vi "Panel Split Engine Example.vi"() -> ()   [LabVIEW 2016]
uses:
  PanelRootNode/PanelRootNode.lvclass
  QueueManager.llb/Destroy.vi
  QueueManager.llb/Remove.vi
  PanelDataNode/PanelDataNode.lvclass
  QueueManager.llb/CreatQueue.vi
  <vilib>/Utility/error.llb/DialogType.ctl
  PanelExample.lvclass
panel:
  out "SelfNode*":refnum<data-value>
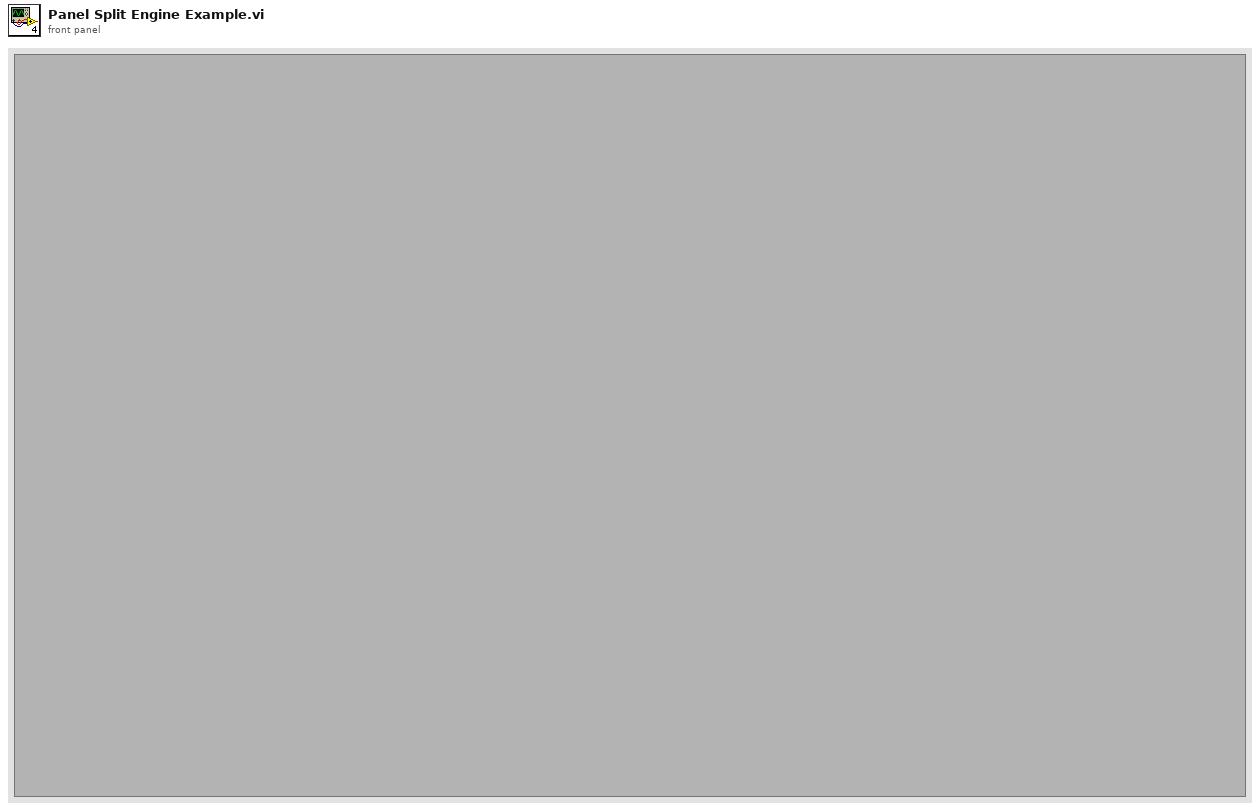
[diagram p1: front panel]
types:
  T1 = cluster{"error":errorcluster, "Event":string, "Data":variant, "Q_Local":string, "RootNode*":refnum<data-value>, "Caller":string}
  T2 = typedef "DialogType.ctl" = u16
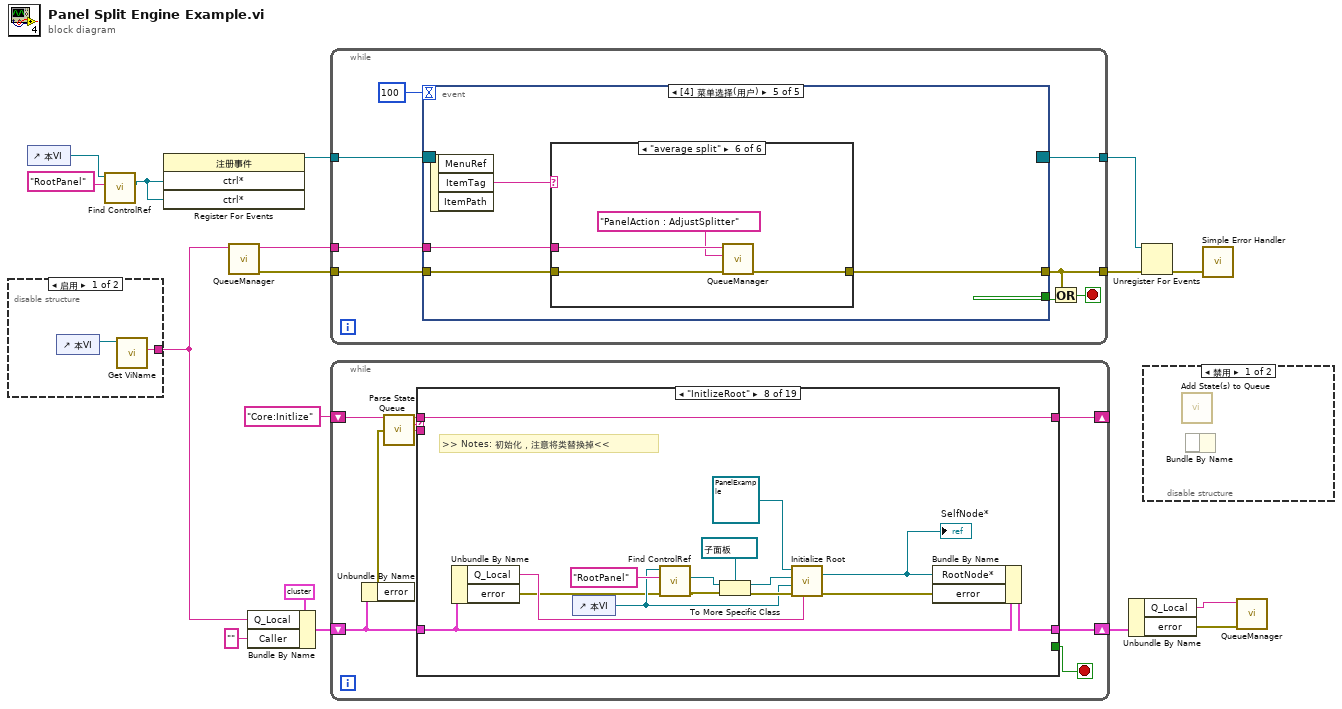
[diagram p0: block diagram]
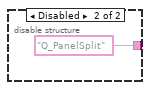
[diagram p2: hidden frame]
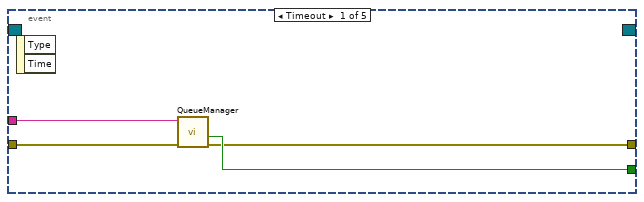
[diagram p4: hidden frame]
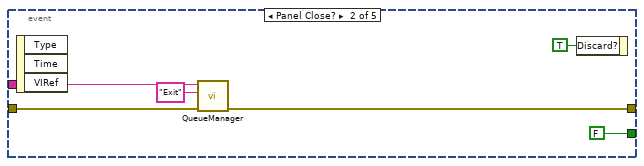
[diagram p5: hidden frame]
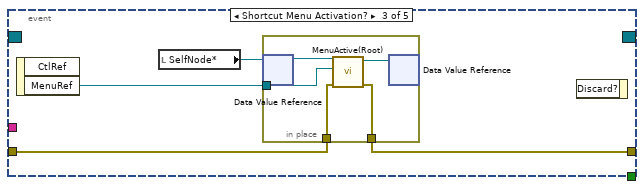
[diagram p6: hidden frame]
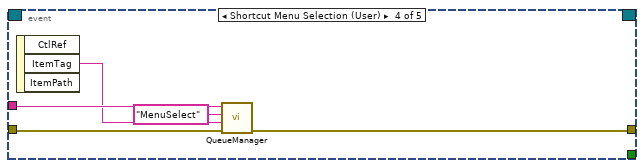
[diagram p7: hidden frame]
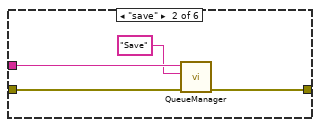
[diagram p9: hidden frame]
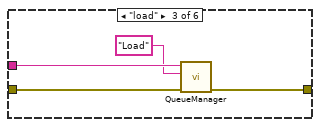
[diagram p10: hidden frame]
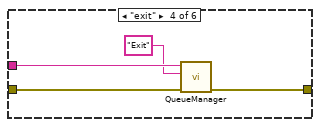
[diagram p11: hidden frame]
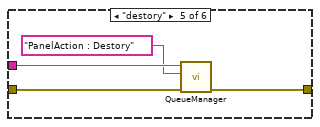
[diagram p12: hidden frame]
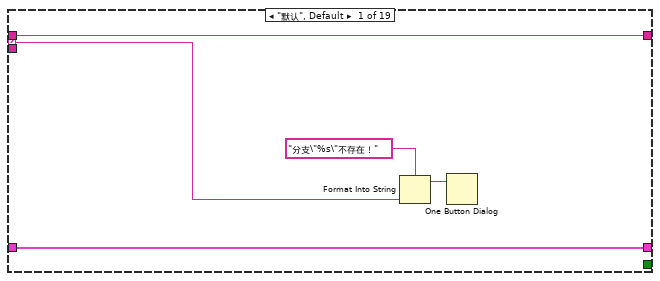
[diagram p13: hidden frame]
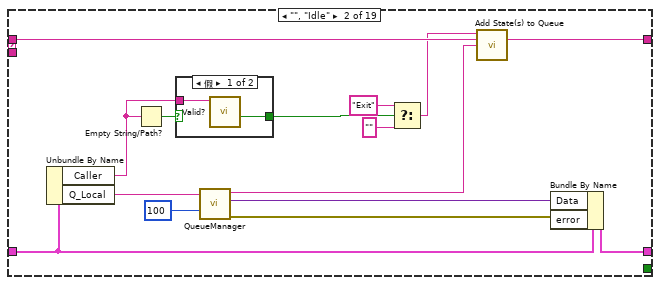
[diagram p14: hidden frame]
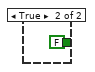
[diagram p15: hidden frame]
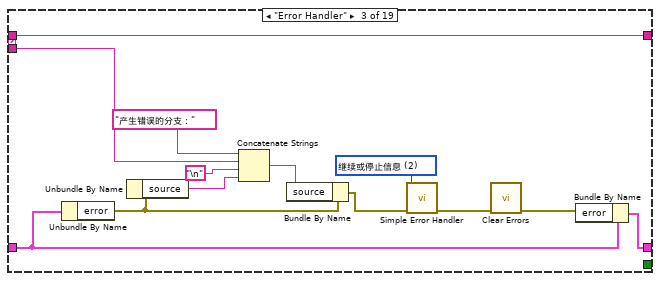
[diagram p16: hidden frame]
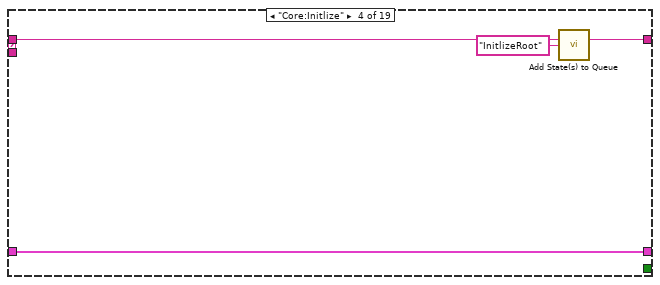
[diagram p17: hidden frame]
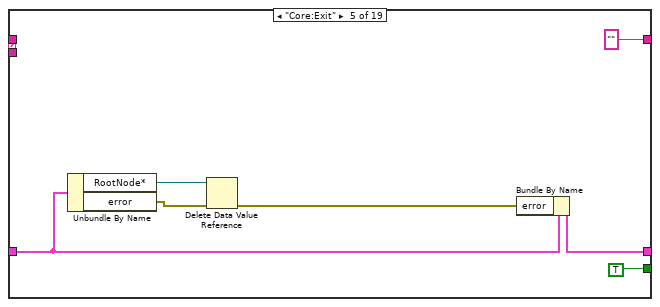
[diagram p18: hidden frame]
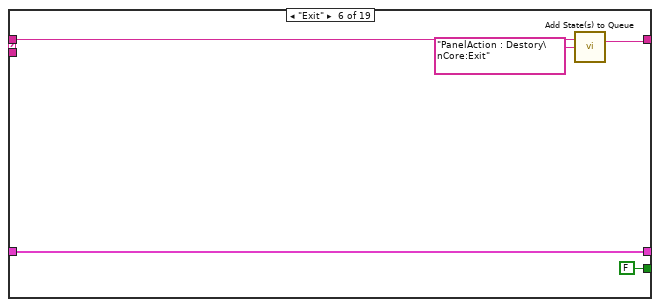
[diagram p19: hidden frame]
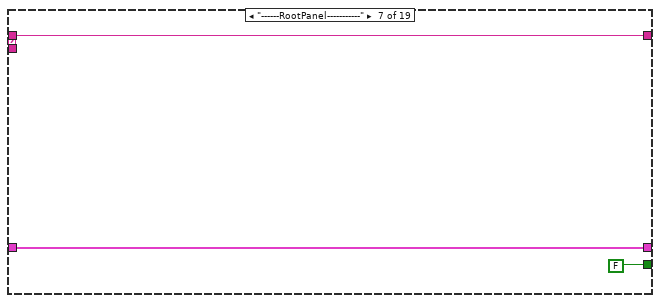
[diagram p20: hidden frame]
diagram:
  n1 = disable-structure shown="启用" {
    disable-tunnel: [w17 "Q_PanelSplit" ("QueueName")] -> w8
    frame Enabled {
      n2 = control-ref of="本VI"() -> (w18:refnum<vi>)
      n3 = call "Get ViName.vi"("VI*"=w18) -> ("VI Name"=w17:string)  [unwired: 8 in, 2 out]
    }
    frame Disabled {
    }
  }
  n4 = control-ref of="本VI"() -> (w6:refnum<vi>)
  n5 = call "Find ControlRef.vi"("control name"="RootPanel", "vi*"=w6) -> ("ctrl*"=w4:refnum<vi>)  [unwired: 7 in, 2 out]
  n6 = register-events(w4, w4) -> (reference out=w9:refnum<event-registration>)  [unwired: 2 in, 1 out]
  n7 = call-poly "QueueManager.vi"("QueueName"=w8) -> ("error out"=w16:errorcluster)  [unwired: 9 in, 1 out]
  n8 = Bundle By Name(cluster=T1 {"error"={"status"=FALSE, "code"=0, "source"=""}, "Event"="", "Data"=variant, "Q_Local"="", "RootNode*"=refnum, "Caller"=""} ("TmpData"), "Q_Local"=w8, "Caller"="") -> (w11:T1)
  n9 = while {
    tunnel: w16 -> [w26]
    tunnel: w8 -> [w27]
    tunnel: [w23] -> w3
    tunnel: w9 -> [w21]
    tunnel: [w20] -> w1
    stop <- w24 stop-if-true
    n10 = event shown="[4] 菜单选择(用户)" {
      selector: w21 -> [_ _ _ _ _]
      dyn-events: [_ _ _ _ _] -> w20
      timeout: 100 -> [_ _ _ _ _]
      tunnel: [w29 FALSE _ _ _] -> w25
      tunnel: w27 -> [w31 w36 _ w51 w54]
      tunnel: w26 -> [w30 w35 w40 w50 w53]
      tunnel: [w28 w34 w41 w49 w52] -> w23
      event Timeout {
        n11 = event-data() -> ()  [unwired: 1 in, 2 out]
        n12 = call-poly "QueueManager.vi"("error in (no error)"=w30, "Queue Name(unamed)"=w31) -> ("error out"=w28:errorcluster, "Not Exist?"=w29:bool)  [unwired: 8 in]
      }
      event Panel Close? {
        n13 = event-data() -> ()  [unwired: 1 in, 3 out]
        n14 = call-poly "QueueManager.vi"("error in"=w35, "Event"="Exit", "QueueName"=w36) -> ("error out"=w34:errorcluster)  [unwired: 7 in, 1 out]
        n15 = event-data("Discard?"=TRUE ("放弃？")) -> ()  [unwired: 1 in, 1 out]
      }
      event Shortcut Menu Activation? {
        n16 = event-data() -> ("MenuRef"=w39:refnum<k9>)  [unwired: 1 in, 1 out]
        n17 = local read "SelfNode*"() -> (w38:refnum<data-value>)
        n18 = in-place {
          in-place-border: w39 -> [w44]
          in-place-border: w40 -> [w43]
          in-place-border: [w42] -> w41
          n19 = in-place-dvr #1(w38) -> (w46:refnum<class "PanelRootNode.lvclass">)  [unwired: 1 out]
          n20 = call "MenuActive(Root).vi"("error in (no error)"=w43, "菜单引用"=w44, "PanelDataNode 输入"=w46) -> ("error out"=w42:errorcluster, "PanelDataNode 输出"=w45:refnum<class "PanelRootNode.lvclass">)  [unwired: 7 in]
          n21 = in-place-dvr #1(w45) -> ()  [unwired: 2 out]
        }
        n22 = event-data() -> ()  [unwired: 2 in, 1 out]
      }
      event Shortcut Menu Selection (User) {
        n23 = event-data() -> ("ItemTag"=w48:string)  [unwired: 1 in, 2 out]
        n24 = call-poly "QueueManager.vi"("error in"=w50, "Data"=w48, "Event"="MenuSelect", "QueueName"=w51) -> ("error out"=w49:errorcluster)  [unwired: 6 in, 1 out]
      }
      event Menu Selection (User) {
        n25 = event-data() -> ("ItemTag"=w55:string)  [unwired: 1 in, 2 out]
        n26 = case shown="\"average split\"" w55 {
          tunnel: w54 -> [_ w60 w64 w68 w72 w76]
          tunnel: w53 -> [w56 w58 w62 w66 w70 w74]
          tunnel: [w56 w57 w61 w65 w69 w73] -> w52
          frame "假", Default {
          }
          frame "save" {
            n27 = call-poly "QueueManager.vi"("error in"=w58, "Event"="Save", "QueueName"=w60) -> ("error out"=w57:errorcluster)  [unwired: 7 in, 1 out]
          }
          frame "load" {
            n28 = call-poly "QueueManager.vi"("error in"=w62, "Event"="Load", "QueueName"=w64) -> ("error out"=w61:errorcluster)  [unwired: 7 in, 1 out]
          }
          frame "exit" {
            n29 = call-poly "QueueManager.vi"("error in"=w66, "Event"="Exit", "QueueName"=w68) -> ("error out"=w65:errorcluster)  [unwired: 7 in, 1 out]
          }
          frame "destory" {
            n30 = call-poly "QueueManager.vi"("error in"=w70, "Event"="PanelAction : Destory", "QueueName"=w72) -> ("error out"=w69:errorcluster)  [unwired: 7 in, 1 out]
          }
          frame "average split" {
            n31 = call-poly "QueueManager.vi"("error in"=w74, "Event"="PanelAction : AdjustSplitter", "QueueName"=w76) -> ("error out"=w73:errorcluster)  [unwired: 7 in, 1 out]
          }
        }
      }
    }
    n32 = Or(x=w23, y=w25) -> (x .or. y?=w24:bool)
  }
  n33 = while {
    shift-right: [w78] -> w13
    shift-left: w11 -> [w79]
    shift-right: [w77] -> _
    shift-left: "Core:Initlize" -> [w85]
    stop <- w81 stop-if-true
    n34 = Unbundle By Name(w79) -> ("error"=w80:errorcluster)
    n35 = call "Parse State Queue.vi"("State Queue"=w85, "Error In (no error)"=w80) -> ("Remaining States"=w84:string, "Current State"=w83:string, "Arguments"=w82:string)  [unwired: 10 in, 1 out]
    n36 = case shown="\"InitlizeRoot\"" w83 {
      selector: w83 -> [w86 _ _ _ _ _ _ _ _ _ _ _ _ _ _ _ _ _ _]
      tunnel: w84 -> [w89 w101 w121 w124 _ w137 w138 w155 w163 w184 w196 w207 w214 w225 w235 w245 w255 w261 w273]
      tunnel: w82 -> [_ _ w109 _ _ _ _ _ _ _ _ _ _ _ _ _ _ _ _]
      tunnel: [_ _ _ _ TRUE FALSE FALSE _ _ _ _ _ _ _ _ _ _ _ _] -> w81
      tunnel: w79 -> [w90 w98 w111 w125 w128 w134 w139 w148 w165 w182 w200 w206 w213 w223 w233 w243 w253 w260 w271]
      tunnel: [w90 w104 w110 w125 w127 w134 w139 w150 w164 w181 w199 w206 w212 w222 w232 w242 w252 w260 w270] -> w78
      tunnel: [w89 w100 w121 w123 "" ("Remaining States") w136 w138 w155 w163 w184 w195 w207 w214 w225 w235 w245 w255 w261 w273] -> w77
      frame "默认", Default {
        n37 = Format Into String(format string="分支\"%s\"不存在！" ("格式字符串"), w86) -> (resulting string=w88:string)  [unwired: 2 in, 1 out]
        n38 = One Button Dialog(message=w88) -> ()  [unwired: 1 in, 1 out]
      }
      frame "", "Idle" {
        n39 = Unbundle By Name(w98) -> ("Caller"=w92:string, "Q_Local"=w97:string)
        n40 = Empty String/Path?(string/path=w92) -> (empty?=w96:bool)
        n41 = case shown="假" w96 {
          tunnel: [w107 FALSE ("Not Exist?")] -> w95
          tunnel: w92 -> [w106 _]
          frame False {
            n42 = call "Valid?.vi"("Queue Name(unamed)"=w106) -> ("Not Exist?"=w107:bool)  [unwired: 9 in, 1 out]
          }
          frame True {
          }
        }
        n43 = call-poly "QueueManager.vi"("Time out(-1)"=100, "Queue Name"=w97) -> ("error out"=w105:errorcluster, "Data"=w103:variant, "Event"=w102:string)  [unwired: 6 in, 1 out]
        n44 = Select(t="Exit" ("Event"), s=w95, f="") -> (s? t:f=w91:string)
        n45 = call "Add State(s) to Queue.vi"("State(s) in Front (\"\")"=w91, "State(s) in (\"\")"=w101, "State(s) at Back (\"\")"=w102) -> ("States Out"=w100:string)  [unwired: 12 in]
        n46 = Bundle By Name(cluster=w98, "Data"=w103, "error"=w105) -> (w104:T1)
      }
      frame "Error Handler" {
        w118 = T2 2 items=["无对话框", "确定信息", "继续或停止信息", "确定信息＋警告", "继续/停止+警告"] ("type of dialog (OK msg:1)")
        n47 = Unbundle By Name(w111) -> ("error"=w113:errorcluster)
        n48 = Unbundle By Name(w113) -> ("source"=w116:string)
        n49 = Concatenate Strings("产生错误的分支：" ("字符串"), w109, "\n", w116) -> (w114:string)
        n50 = Bundle By Name(cluster=w113, "source"=w114) -> (w112:errorcluster)
        n51 = call <vilib>:"Simple Error Handler.vi"("type of dialog (OK msg:1)"=w118, "error in (no error)"=w112) -> ("error out"=w119:errorcluster)  [unwired: 3 in, 4 out]
        n52 = call <vilib>:"Clear Errors.vi"("error in (no error)"=w119) -> ("error out"=w120:errorcluster)  [unwired: 5 in, 1 out]
        n53 = Bundle By Name(cluster=w111, "error"=w120) -> (w110:T1)
      }
      frame "Core:Initlize" {
        n54 = call "Add State(s) to Queue.vi"("State(s) in (\"\")"=w124, "State(s) at Back (\"\")"="InitlizeRoot" ("State(s) at Back (\"\")")) -> ("States Out"=w123:string)  [unwired: 13 in]
      }
      frame "Core:Exit" {
        n55 = Unbundle By Name(w128) -> ("RootNode*"=w130:refnum<data-value>, "error"=w126:errorcluster)
        n56 = Delete Data Value Reference(data value reference=w130, error in=w126) -> (error out=w129:errorcluster)  [unwired: 1 out]
        n57 = Bundle By Name(cluster=w128, "error"=w129) -> (w127:T1)
      }
      frame "Exit" {
        n58 = call "Add State(s) to Queue.vi"("State(s) in (\"\")"=w137, "State(s) at Back (\"\")"="PanelAction : Destory\nCore:Exit" ("State(s) at Back (\"\")")) -> ("States Out"=w136:string)  [unwired: 13 in]
      }
      frame "------RootPanel-----------" {
      }
      frame "InitlizeRoot" {
        # ">> Notes: 初始化，注意将类替换掉<<"
        n59 = Unbundle By Name(w148) -> ("Q_Local"=w147:string, "error"=w142:errorcluster)
        n60 = control-ref of="本VI"() -> (w143:refnum<vi>)
        n61 = call "Find ControlRef.vi"("error in (no error)"=w142, "control name"="RootPanel", "vi*"=w143) -> ("error out"=w145:errorcluster, "ctrl*"=w144:refnum<vi>)  [unwired: 6 in, 1 out]
        n62 = To More Specific Class(target class=refnum<vi> refnum ("RootPanel"), reference=w144, error in=w145) -> (specific class reference=w153:refnum<vi>, error out=w152:errorcluster)
        n63 = call-dynamic "Initialize Root.vi"("RootQueueName"=w147, "error in (no error)"=w152, "CurrentVi*"=w143, "RootPanel*"=w153, "PanelRootNode 输入"=refnum<class "PanelExample.lvclass"> refnum ("PanelExample.lvclass")) -> ("error out"=w151:errorcluster, "SelfNode*"=w149:refnum<data-value>)  [unwired: 5 in]
        "SelfNode*" <- w149
        n64 = Bundle By Name(cluster=w148, "RootNode*"=w149, "error"=w151) -> (w150:T1)
      }
      frame "Save" {
        # ">> Notes: 保存分割结果，可通过队列发送保存的路径，也可不发送路径，自动弹出文件选择对话框。<<"
        n65 = Unbundle By Name(w165) -> ("RootNode*"=w166:refnum<data-value>, "Data"=w161:variant, "error"=w156:errorcluster)
        n66 = Variant To Data(error in=w156, type=path "" ("路径"), Variant=w161) -> (data=w159:path, error out=w158:errorcluster)
        n67 = call <vilib>:"Clear Errors.vi"("error in (no error)"=w158) -> ("error out"=w157:errorcluster)  [unwired: 5 in, 1 out]
        n68 = in-place {
          in-place-border: [w169] -> w162
          in-place-border: w159 -> [w168]
          in-place-border: w157 -> [w167]
          n69 = in-place-dvr #2(w166) -> (w171:refnum<class "PanelRootNode.lvclass">)  [unwired: 1 out]
          n70 = call-dynamic "Save Xml.vi"("error in"=w167, "selected path"=w168, "PanelRootNode 输入"=w171) -> ("error out"=w169:errorcluster, "PanelRootNode 输出"=w170:refnum<class "PanelRootNode.lvclass">)  [unwired: 7 in]
          n71 = in-place-dvr #2(w170) -> ()  [unwired: 2 out]
        }
        n72 = Bundle By Name(cluster=w165, "error"=w162) -> (w164:T1)
      }
      frame "Load" {
        n73 = Unbundle By Name(w182) -> ("RootNode*"=w183:refnum<data-value>, "Data"=w178:variant, "error"=w175:errorcluster)
        n74 = Variant To Data(error in=w175, type=path "" ("路径"), Variant=w178) -> (data=w177:path, error out=w179:errorcluster)
        n75 = call <vilib>:"Clear Errors.vi"("error in (no error)"=w179) -> ("error out"=w176:errorcluster)  [unwired: 5 in, 1 out]
        n76 = in-place {
          in-place-border: [w188] -> w173
          in-place-border: w177 -> [w186]
          in-place-border: w176 -> [w185]
          n77 = in-place-dvr #3(w183) -> (w187:refnum<class "PanelRootNode.lvclass">)  [unwired: 1 out]
          n78 = call-dynamic "Load Xml.vi"("error in"=w185, "selected path"=w186, "PanelRootNode 输入"=w187) -> ("error out"=w188:errorcluster, "PanelRootNode 输出"=w189:refnum<class "PanelRootNode.lvclass">)  [unwired: 7 in]
          n79 = in-place-dvr #3(w189) -> (w174:errorcluster)  [unwired: 1 out]
        }
        n80 = Merge Errors(w174, w173) -> (w172:errorcluster)
        n81 = Bundle By Name(cluster=w182, "error"=w172) -> (w181:T1)
      }
      frame "MenuSelect" {
        n82 = Unbundle By Name(w200) -> ("RootNode*"=w194:refnum<data-value>, "Data"=w198:variant, "error"=w190:errorcluster)
        n83 = Variant To Data(error in=w190, type="", Variant=w198) -> (data=w193:string, error out=w192:errorcluster)
        n84 = in-place {
          in-place-border: w193 -> [w203]
          in-place-border: w192 -> [w202]
          in-place-border: [w201] -> w191
          n85 = in-place-dvr #4(w194) -> (w205:refnum<class "PanelRootNode.lvclass">)  [unwired: 1 out]
          n86 = call-dynamic "MenuSelect.vi"("error in"=w202, "Tag"=w203, "PanelRootNode 输入"=w205) -> ("error out"=w201:errorcluster, "PanelRootNode 输出"=w204:refnum<class "PanelRootNode.lvclass">)  [unwired: 7 in]
          n87 = in-place-dvr #4(w204) -> ()  [unwired: 2 out]
        }
        n88 = Bundle By Name(cluster=w200, "error"=w191) -> (w199:T1)
        n89 = call "Add State(s) to Queue.vi"("State(s) in (\"\")"=w196) -> ("States Out"=w195:string)  [unwired: 14 in]
      }
      frame "-------PanelAction----------" {
      }
      frame "PanelAction : Split" {
        n90 = Unbundle By Name(w213) -> ("RootNode*"=w211:refnum<data-value>, "Data"=w210:variant, "error"=w208:errorcluster)
        n91 = in-place {
          in-place-border: w210 -> [w217]
          in-place-border: [w216] -> w209
          in-place-border: w208 -> [w215]
          n92 = in-place-dvr #5(w211) -> (w219:refnum<class "PanelRootNode.lvclass">)  [unwired: 1 out]
          n93 = call-dynamic "Split.vi"("error in"=w215, "Data"=w217, "PanelRootNode 输入"=w219) -> ("error out"=w216:errorcluster, "PanelRootNode 输出"=w218:refnum<class "PanelRootNode.lvclass">)  [unwired: 7 in]
          n94 = in-place-dvr #5(w218) -> ()  [unwired: 2 out]
        }
        n95 = Bundle By Name(cluster=w213, "error"=w209) -> (w212:T1)
      }
      frame "PanelAction : Delete" {
        n96 = Unbundle By Name(w223) -> ("RootNode*"=w224:refnum<data-value>, "Data"=w221:variant)
        n97 = in-place {
          in-place-border: w221 -> [w227]
          in-place-border: [w226] -> w220
          n98 = in-place-dvr #6(w224) -> (w229:refnum<class "PanelRootNode.lvclass">)  [unwired: 1 out]
          n99 = call-dynamic "Delete.vi"("Data"=w227, "PanelRootNode 输入"=w229) -> ("error out"=w226:errorcluster, "PanelRootNode 输出"=w228:refnum<class "PanelRootNode.lvclass">)  [unwired: 8 in]
          n100 = in-place-dvr #6(w228) -> ()  [unwired: 2 out]
        }
        n101 = Bundle By Name(cluster=w223, "error"=w220) -> (w222:T1)
      }
      frame "PanelAction : Insert" {
        n102 = Unbundle By Name(w233) -> ("RootNode*"=w234:refnum<data-value>, "Data"=w230:variant)
        n103 = in-place {
          in-place-border: [w236] -> w231
          in-place-border: w230 -> [w237]
          n104 = in-place-dvr #7(w234) -> (w239:refnum<class "PanelRootNode.lvclass">)  [unwired: 1 out]
          n105 = call-dynamic "Insert.vi"("Data"=w237, "PanelRootNode 输入"=w239) -> ("error out"=w236:errorcluster, "PanelRootNode 输出"=w238:refnum<class "PanelRootNode.lvclass">)  [unwired: 8 in]
          n106 = in-place-dvr #7(w238) -> ()  [unwired: 2 out]
        }
        n107 = Bundle By Name(cluster=w233, "error"=w231) -> (w232:T1)
      }
      frame "PanelAction : Destory" {
        # ">> Notes: 销毁分割结果，回到最初状态<<"
        n108 = Unbundle By Name(w243) -> ("RootNode*"=w244:refnum<data-value>, "error"=w240:errorcluster)
        n109 = in-place {
          in-place-border: [w247] -> w241
          in-place-border: w240 -> [w246]
          n110 = in-place-dvr #8(w244) -> (w249:refnum<class "PanelRootNode.lvclass">)  [unwired: 1 out]
          n111 = call-dynamic "Destory.vi"("error in (no error)"=w246, "PanelRootNode 输入"=w249) -> ("error out"=w247:errorcluster, "PanelRootNode 输出"=w248:refnum<class "PanelRootNode.lvclass">)  [unwired: 8 in]
          n112 = in-place-dvr #8(w248) -> ()  [unwired: 2 out]
        }
        n113 = Bundle By Name(cluster=w243, "error"=w241) -> (w242:T1)
      }
      frame "PanelAction : AdjustSplitter" {
        # ">> Notes: 均分面板<<"
        n114 = Unbundle By Name(w253) -> ("RootNode*"=w254:refnum<data-value>, "error"=w250:errorcluster)
        n115 = in-place {
          in-place-border: [w257] -> w251
          in-place-border: w250 -> [w256]
          n116 = in-place-dvr #9(w254) -> (w259:refnum<class "PanelRootNode.lvclass">)  [unwired: 1 out]
          n117 = call "Adjust Splitter.vi"("error in (no error)"=w256, "PanelRootNode 输入"=w259) -> ("error out"=w257:errorcluster, "PanelRootNode 输出"=w258:refnum<class "PanelRootNode.lvclass">)  [unwired: 8 in]
          n118 = in-place-dvr #9(w258) -> ()  [unwired: 2 out]
        }
        n119 = Bundle By Name(cluster=w253, "error"=w251) -> (w252:T1)
      }
      frame "------Communication---------" {
      }
      frame "SendToAll" {
        # ">> Notes: 发送至所有面板中插入的VI线程，要求插入的VI使用的队列名是VI名称；<<"
        n120 = Unbundle By Name(w271) -> ("RootNode*"=w272:refnum<data-value>, "Data"=w268:variant, "error"=w262:errorcluster)
        n121 = Variant To Data(error in=w262, type=cluster{"Event":string, "Data":variant} {"Event"="", "Data"=variant}, Variant=w268) -> (data=w266:cluster{"Event":string, "Data":variant}, error out=w263:errorcluster)
        n122 = Unbundle By Name(w266) -> ("Event"=w265:string, "Data"=w264:variant)
        n123 = in-place {
          in-place-border: [w278] -> w269
          in-place-border: w265 -> [w277]
          in-place-border: w264 -> [w276]
          in-place-border: w263 -> [w275]
          n124 = in-place-dvr #10(w272) -> (w280:refnum<class "PanelRootNode.lvclass">)  [unwired: 1 out]
          n125 = call "SendToPanels.vi"("PanelNumber(-1)"=-1, "error in"=w275, "Data"=w276, "Event"=w277, "PanelRootNode in"=w280) -> ("error out"=w278:errorcluster, "PanelRootNode out"=w279:refnum<class "PanelRootNode.lvclass">)  [unwired: 5 in]
          n126 = in-place-dvr #10(w279) -> ()  [unwired: 2 out]
        }
        n127 = Bundle By Name(cluster=w271, "error"=w269) -> (w270:T1)
      }
    }
  }
  n128 = Unbundle By Name(w13) -> ("Q_Local"=w10:string, "error"=w14:errorcluster)
  n129 = Unregister For Events(event registration refnum=w1, error in=w3) -> (error out=w2:errorcluster)
  n130 = disable-structure shown="禁用" {
    frame Disabled {
      n131 = call "Add State(s) to Queue.vi"() -> ()  [unwired: 15 in, 1 out]
      n132 = Bundle By Name() -> ()  [unwired: 2 in, 1 out]
    }
    frame Enabled {
    }
  }
  n133 = call <vilib>:"Simple Error Handler.vi"("error in (no error)"=w2) -> ()  [unwired: 4 in, 5 out]
  n134 = call-poly "QueueManager.vi"("error in (no error)"=w14, "QueeuName"=w10) -> ()  [unwired: 9 in, 1 out]
